vi "SR7265 VoscVxVy Read_DP_ver1.0.vi"(0 "GPIB ADR":i16, 3 "error in":errorcluster) -> (1 "Vosc (volt)":dbl, 5 "Vx (volt)":dbl, 6 "dump GPIB ADR":i16, 7 "Vy (volt)":dbl, 9 "error out":errorcluster)   [LabVIEW 2012]
doc: "SR7265 Vos , Vx, and Vy Read out"
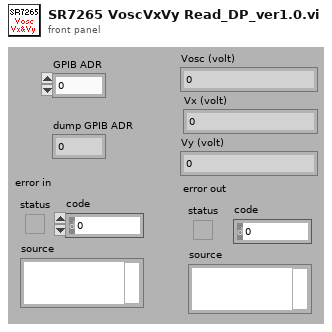
[diagram p1: front panel]
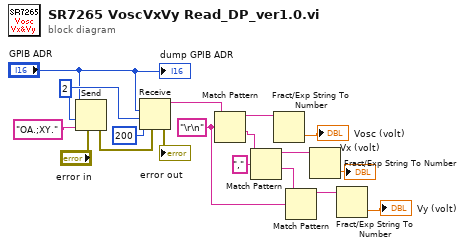
[diagram p0: block diagram]
diagram:
  w6 = "\r\n" ("regular expression")
  w15 = i16 2 ("mode")
  n1 = Send(2:"GPIB ADR", 3:w15, 4:"error in", 5:"OA.;XY." ("data string")) -> (8:w14:errorcluster)  [unwired: 1 in, 2 out]
  n2 = Receive(4:w14, 6:200 ("count"), 7:w15, 8:"GPIB ADR") -> (0:→"error out":errorcluster, 3:w5:string)  [unwired: 1 in, 2 out]
  n3 = Match Pattern(string=w5, regular expression=w6) -> (before substring=w3:string, after substring=w8:string)  [unwired: 1 in, 2 out]
  n4 = Match Pattern(string=w8, regular expression=",") -> (before substring=w2:string, after substring=w7:string)  [unwired: 1 in, 2 out]
  n5 = Fract/Exp String To Number(string=w3) -> (number=→"Vosc (volt)":dbl)  [unwired: 3 in, 1 out]
  n6 = Match Pattern(string=w7, regular expression=w6) -> (before substring=w1:string)  [unwired: 1 in, 3 out]
  n7 = Fract/Exp String To Number(string=w2) -> (number=→"Vx (volt)":dbl)  [unwired: 3 in, 1 out]
  n8 = Fract/Exp String To Number(string=w1) -> (number=→"Vy (volt)":dbl)  [unwired: 3 in, 1 out]
  "dump GPIB ADR" <- "GPIB ADR"
